vi "TerrainAuto.vi"(8 "error in (no error)":errorcluster) -> ()   [LabVIEW 2015]
uses:
  Utilities/MotorPositionGlobals.vi
  Utilities/JoystickGlobals.vi
panel:
  in  "JoystickValues":dbl[](array[numeric])
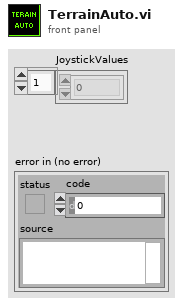
[diagram p1: front panel]
types:
  T1 = typedef "WPI_MotorControlDeviceRef.ctl" = cluster{"DeviceStatus":errorcluster, "Type":T2, "PWM":cluster{"PWM Channel":T3, "DeadBand":T4}, "CAN":cluster{"Device Number":u8, "Control Mode":T5, "Semaphore":T6, "Max Vout":dbl, "TalonSRX Control Mode":T7}, "Invert":bool}
  T2 = typedef "WPI_MotorControlType.ctl" = enum16{"PWM", "CAN", "CANTalonSRX"}
  T3 = typedef "FPGA_DIOPWMChannel.ctl" = enum8{"PWM 0", "PWM 1", "PWM 2", "PWM 3", "PWM 4", "PWM 5", "PWM 6", "PWM 7", "PWM 8", "PWM 9", "PWM MXP 0", "PWM MXP 1", "PWM MXP 2", "PWM MXP 3", "PWM MXP 4", "PWM MXP 5", "PWM MXP 6", "PWM MXP 7", "PWM MXP 8", "PWM MXP 9", "Invalid"}
  T4 = typedef "WPI_PWMDeadband.ctl" = cluster{"Name":string, "maxPositivePwm":i32, "minPositivePwm":i32, "centerPwm":i32, "maxNegativePwm":i32, "minNegativePwm":i32, "angularRange":u16}
  T5 = typedef "WPI_CANJaguar_ControlMode.ctl" = enum8{"Percent VBus", "Current", "Speed", "Position", "Voltage"}
  T6 = typedef "Semaphore RefNum" = refnum<k1>
  T7 = typedef "WPI_CANTalonSRX_APIControlMode.ctl" = enum8{"Percent VBus", "Speed", "Position", "Slave", "Unchanged / Invalid", "Voltage Compensation", "Current", "Motion Profile"}
  T8 = typedef "WPI_CANTalonSRX_GlobalStatus.ctl" = cluster{"Applied Throttle":dbl, "Module Enabled":bool, "CAN Error":errorcluster, "Closed Loop Error":dbl, "Forward Limit Switch Closed":bool, "Reverse Limit Switch Closed":bool, "Sensor Position":dbl, "Sensor Velocity":dbl, "Current":dbl, "Sticky Fault - Over Temp":bool, "Sticky Fault - Under Voltage":bool, "Sticky Fault - Forward Limit":bool, "Sticky Fault - Reverse Limit":bool, "Sticky Fault - Forward Soft Limit":bool, "Sticky Fault - Reverse Soft Limit":bool, "Brake is Enabled":bool, "Encoder Position":dbl, "Encoder Velocity":dbl, "Encoder Index Count":dbl, "Encoder A Pin State":bool, "Encoder B Pin State":bool, "Encoder Index Pin State":bool, "Analog In":dbl, "Analog In Velocity":dbl, "Temperature (C)":dbl, "Battery Voltage":dbl, "Control 5 Is Supported":bool, "Current Profile Slot Select":dbl, "Pos Div 8":bool, "Vel Div 4":bool, "Pulse Width Position":i32, "Pulse Width Velocity":i32, "Pulse Width Rise To Rise (us)":i32, "Pulse Width Rise To Fall (us)":i32, "Mot Prof Active Is Under Run":bool, "Mot Prof Active Has Under Run":bool, "Mot Prof Active Is Last":bool, "Mot Prof Active Velocity Only":bool, "Mot Prof Active Is Valid":bool, "Mot Prof Buffer Is Full":bool, "Mot Prof Active Profile Slot Select":i32, "Mot Prof NextID":i32, "Mot Prof Count":i32, "Mot Prof Active Velocity":dbl, "Mot Prof Active Position":dbl, "Mot Prof Output Enable":i32}
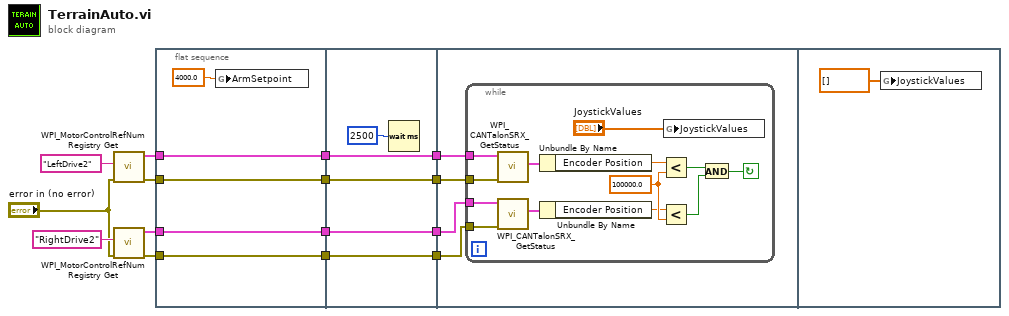
[diagram p0: block diagram]
diagram:
  n1 = call <vilib>:"WPI_MotorControlRefNum Registry Get.vi"("error in (no error)"="error in (no error)", "refnum name"="LeftDrive2") -> ("error out"=w9:errorcluster, "MotorControlDevRef"=w12:T1)  [unwired: 8 in]
  n2 = call <vilib>:"WPI_MotorControlRefNum Registry Get.vi"("error in (no error)"="error in (no error)", "refnum name"="RightDrive2") -> ("error out"=w3:errorcluster, "MotorControlDevRef"=w6:T1)  [unwired: 8 in]
  n3 = flat-sequence {
    tunnel: w12 -> [w19]
    tunnel: [w19] -> w10
    tunnel: w9 -> [w18]
    tunnel: [w18] -> w7
    tunnel: w6 -> [w17]
    tunnel: [w17] -> w4
    tunnel: w3 -> [w16]
    tunnel: [w16] -> w1
    tunnel: [w24] -> w11
    tunnel: w10 -> [w24]
    tunnel: [w23] -> w8
    tunnel: w7 -> [w23]
    tunnel: [w22] -> w5
    tunnel: w4 -> [w22]
    tunnel: [w21] -> w2
    tunnel: w1 -> [w21]
    tunnel: w11 -> [w29]
    tunnel: w8 -> [w28]
    tunnel: w5 -> [w27]
    tunnel: w2 -> [w26]
    frame #0 {
      n4 = global write "MotorPositionGlobals.vi" "ArmSetpoint"(4000.0 ("ArmSetpoint")) -> ()
    }
    frame #1 {
      n5 = Wait (ms)(milliseconds to wait=u32 2500) -> ()  [unwired: 1 out]
    }
    frame #2 {
      n6 = while {
        tunnel: w29 -> [w34]
        tunnel: w28 -> [w33]
        tunnel: w27 -> [w32]
        tunnel: w26 -> [w31]
        stop <- w30 continue-if-true
        w39 = 100000.0 ("y")
        n7 = call <vilib>:"WPI_CANTalonSRX_GetStatus.vi"("error in (no error)"=w33, "CAN Talon SRX Ref"=w34) -> ("Talon SRX Status"=w35:T8)  [unwired: 7 in, 2 out]
        n8 = call <vilib>:"WPI_CANTalonSRX_GetStatus.vi"("error in (no error)"=w31, "CAN Talon SRX Ref"=w32) -> ("Talon SRX Status"=w36:T8)  [unwired: 7 in, 2 out]
        n9 = Unbundle By Name(w35) -> ("Encoder Position"=w37:dbl)
        n10 = Unbundle By Name(w36) -> ("Encoder Position"=w38:dbl)
        n11 = Less?(x=w37, y=w39) -> (x < y?=w41:bool)
        n12 = Less?(x=w38, y=w39) -> (x < y?=w40:bool)
        n13 = global write "JoystickGlobals.vi" "JoystickValues"("JoystickValues") -> ()
        n14 = And(x=w41, y=w40) -> (x .and. y?=w30:bool)
      }
    }
    frame #3 {
      n15 = global write "JoystickGlobals.vi" "JoystickValues"(dbl[] [] ("JoystickValues")) -> ()
    }
  }
